vi "Tone.vi"(7 "Duration (20 ms)":u32=20, 8 "Error In":errorcluster, 9 "Frequency (0 Hz)":u16 step=100, 10 "Buzzer Pin":u8=8, 11 "ChipKit Resource":T1={"COM Port"="", "Board Type"=enum."ChipKit uC32", "Connection Type"=enum."USB / Serial", "Baud Rate (115200)"=15, "Bytes Per Packet (15)"=15}) -> (0 "Error Out":errorcluster, 3 "ChipKit Resource":T1={"COM Port"="", "Board Type"=enum."ChipKit uC32", "Connection Type"=enum."USB / Serial", "Baud Rate (115200)"=15, "Bytes Per Packet (15)"=15})   [LabVIEW 2011, in "LabVIEW Interface for ChipKit.lvlib"]
doc: "Generates a square wave with the specified frequency and 50% duty cycle. Use this VI with frequency equal to 0 to stop the signal generation on the specified pin. This command can only be used on one pin at a time and signal generation must be stopped on one pin before it can be started on another."
uses:
  LabVIEW Interface for ChipKit.lvlib
  Private/Type Defs/Chipkit Resource.ctl
  Private/Type Defs/Board Type.ctl
  Private/Type Defs/Connection Type.ctl
  Private/Type Defs/Command.ctl
  Private/Type Defs/Pin Type.ctl
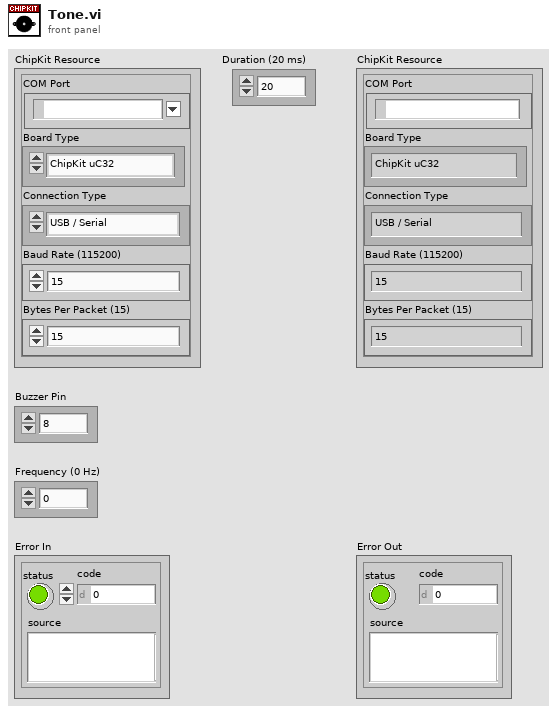
[diagram p1: front panel]
types:
  T1 = typedef "LabVIEW Interface for ChipKit.lvlib/Chipkit Resource.ctl" = cluster{"COM Port":refnum<visa-resource-name>, "Board Type":T2, "Connection Type":T3, "Baud Rate (115200)":u32, "Bytes Per Packet (15)":u32}
  T2 = typedef "LabVIEW Interface for ChipKit.lvlib/Board Type.ctl" = enum16{"ChipKit uC32", "ChipKit Uno32", "ChipKit Max32"}
  T3 = typedef "LabVIEW Interface for ChipKit.lvlib/Connection Type.ctl" = enum8{"USB / Serial", "XBEE", "BlueSmirf (Bluetooth)"}
  T4 = typedef "LabVIEW Interface for ChipKit.lvlib/Pin Type.ctl" = enum8{"Analog", "Digital", "PWM", "Tone"}
  T5 = typedef "LabVIEW Interface for ChipKit.lvlib/Command.ctl" = enum8{"setArduinoMode", "flushSerial", "setPinMode", "digitalWritePin", "digitalWritePort", "tone", "digitalReadPin", "digitalReadPort", "analogReadPin", "analogReadPort", "pwmWritePin", "pwmWritePort", "sevenSegment_Configure", "sevenSegment_Write", "I2C Init", "I2C Write", "I2C Read", "SPI Init", "SPI Set Bit Order", "SPI Set Clock Divider", "SPI Set Data Mode", "SPI Send / Receive", "SPI Close", "Servo Set Num Servos", "Servo Config Servo", "Servo Write Angle", "Servo Read Angle", "Servo Write Pulse Width", "Servo Read Pulse Width", "Servo Detach", "LCD Init", "LCD Set Size", "LCD Set Cursor Mode", "LCD Clear", "LCD Set Cursor Position", "LCD Print", "LCD Display Power", "LCD Scroll Display", "LCD Autoscroll", "LCD Print Direction", "LCD Create Custom Char", "LCD Print Custom Char", "contAcqOn", "contAcqOff", "getFirmwareVersion", "FiniteSampleStart", "NA", "NA2", "Conifg Stepper", "Stepper Write", "Stepper Detach", "Stepper Steps To Go", "Config DO Port", "Config DI Port", "UART2 Open", "UART2 Write", "UART2 Bytes Available", "UART2 Read"}
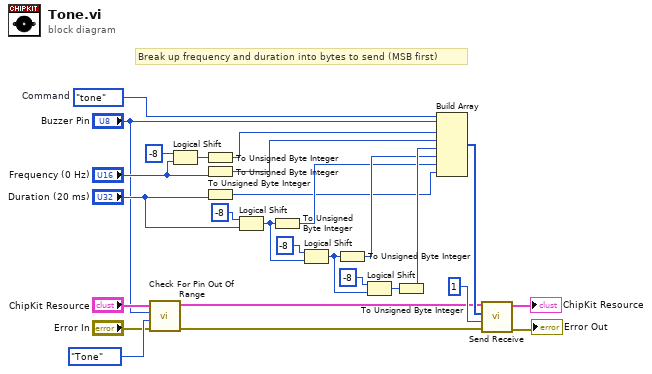
[diagram p0: block diagram]
diagram:
  w7 = Command."tone"  # Command
  # "Break up frequency and duration into bytes to send (MSB first)"
  n1 = call "Check For Pin Out Of Range.vi"("Error In"="Error In", "Pin Type"=Pin_Type."Tone", "User Pin Number"="Buzzer Pin", "Arduino Resource"="ChipKit Resource") -> ("Error Out"=w2:errorcluster, "Arduino Resource"=w4:T1)  [unwired: 6 in]
  n2 = Logical Shift(y=i8 -8, x="Frequency (0 Hz)") -> (x << y=w12:u16)
  n3 = To Unsigned Byte Integer(number=w12) -> (unsigned 8bit integer=w13:u8)
  n4 = To Unsigned Byte Integer(number="Frequency (0 Hz)") -> (unsigned 8bit integer=w10:u8)
  n5 = To Unsigned Byte Integer(number="Duration (20 ms)") -> (unsigned 8bit integer=w15:u8)
  n6 = Logical Shift(y=i8 -8, x="Duration (20 ms)") -> (x << y=w20:u32)
  n7 = To Unsigned Byte Integer(number=w20) -> (unsigned 8bit integer=w16:u8)
  n8 = Logical Shift(y=i8 -8, x=w20) -> (x << y=w21:u32)
  n9 = To Unsigned Byte Integer(number=w21) -> (unsigned 8bit integer=w22:u8)
  n10 = Logical Shift(y=i8 -8, x=w21) -> (x << y=w19:u32)
  n11 = To Unsigned Byte Integer(number=w19) -> (unsigned 8bit integer=w23:u8)
  n12 = Build Array(w7, "Buzzer Pin", w13, w10, w23, w22, w16, w15) -> (w24:u8[])
  n13 = call "Send Receive.vi"("Error In"=w2, "Bytes To Read (0)"=u8 1, "Data"=w24, "ChipKit Resource"=w4) -> ("Error Out"=→"Error Out":errorcluster, "ChipKit Resource"=→"ChipKit Resource":T1)  [unwired: 5 in, 1 out]
